vi "G4BaseTemplate_Singleton_4x4x4_ReadAttribute.vi"(8 "Error In":errorcluster) -> (0 "Error Out":errorcluster)   [LabVIEW 2020]
uses:
  <resource>/Framework/Providers/Open_GDS/ClassProviders/Provider_EndevoGOOP400/Templates/G4BaseTemplate_Singleton_4x4x4/G4BaseTemplate_Singleton_4x4x4.lvclass
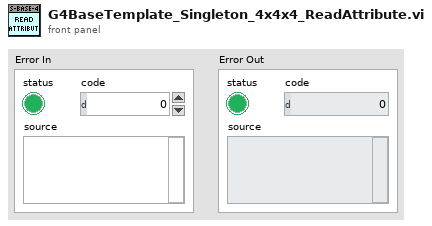
[diagram p1: front panel]
types:
  T1 = typedef "G4BaseTemplate_Singleton_4x4x4.lvclass/ObjectAttributes.ctl" = cluster{"Attribute1":dbl}
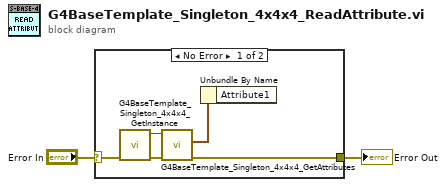
[diagram p0: block diagram]
diagram:
  n1 = case shown="No Error" "Error In" {
    selector: "Error In" -> [w4 w8]
    tunnel: [w6 w8] -> w1
    frame No Error {
      n2 = call <resource>:"G4BaseTemplate_Singleton_4x4x4_GetInstance.vi"("error in (no error)"=w4) -> ("error out"=w3:errorcluster, "reference out"=w5:refnum<class "G4BaseTemplate_Singleton_4x4x4.lvclass">)  [unwired: 6 in, 3 out]
      n3 = call <resource>:"G4BaseTemplate_Singleton_4x4x4_GetAttributes.vi"("error in (no error)"=w3, "reference in"=w5) -> ("error out"=w6:errorcluster, "Data"=w7:T1)  [unwired: 6 in, 2 out]
      n4 = Unbundle By Name(w7) -> ()  [unwired: 1 out]
    }
    frame Error {
    }
  }
  "Error Out" <- w1
